vi "Write Message queue.vi"(8 "error in (no error)":errorcluster, 10 "Message queue":refnum<queue>, 11 "Parent Actor in":refnum<class "Parent Actor.lvclass">) -> (0 "error out":errorcluster, 3 "Parent Actor out":refnum<class "Parent Actor.lvclass">)   [LabVIEW 2015, in "Parent Actor.lvclass"]
uses:
  Parent Actor.lvclass
  Parent Message/Parent Message.lvclass
  Parent Actor.lvclass/Parent Actor.ctl
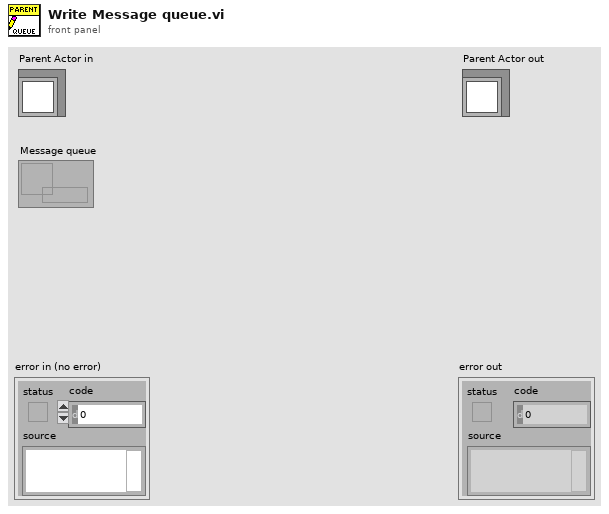
[diagram p1: front panel]
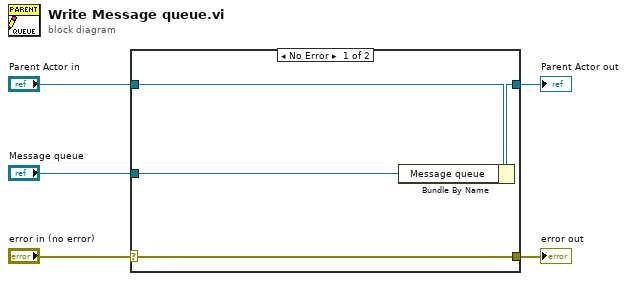
[diagram p0: block diagram]
diagram:
  n1 = case shown="No Error" "error in (no error)" {
    selector: "error in (no error)" -> [w9 w10]
    tunnel: [w9 w10] -> w4
    tunnel: [w7 w11] -> w2
    tunnel: "Parent Actor in" -> [w8 w11]
    tunnel: "Message queue" -> [w6 _]
    frame No Error {
      n2 = Bundle By Name(cluster=w8, "Message queue"=w6) -> (w7:refnum<class "Parent Actor.lvclass">)
    }
    frame Error {
    }
  }
  "error out" <- w4
  "Parent Actor out" <- w2
